vi "ZCAN_FilterClear.vi"(0 "error in (no error)":errorcluster caption="错误输入（无错误）", 2 "can_index_handle":u32, 5 "can_index":u32) -> (14 "error out":errorcluster caption="错误输出", 16 "can_index_handle(out)":u32, 19 "can_index(out)":u32)   [LabVIEW 2020, in "zlgcan.lvlib"]
uses:
  zlgcan.lvlib
  bin/zlgcan_wrap.dll
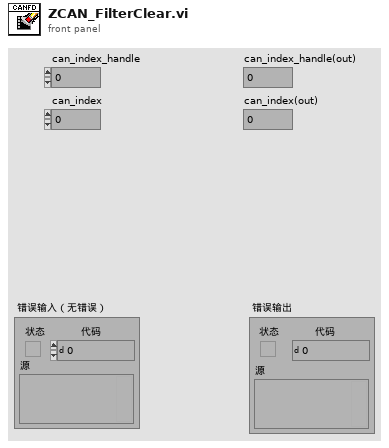
[diagram p1: front panel]
types:
  T1 = cluster{"status":bool, "return":u32, "消息":string}
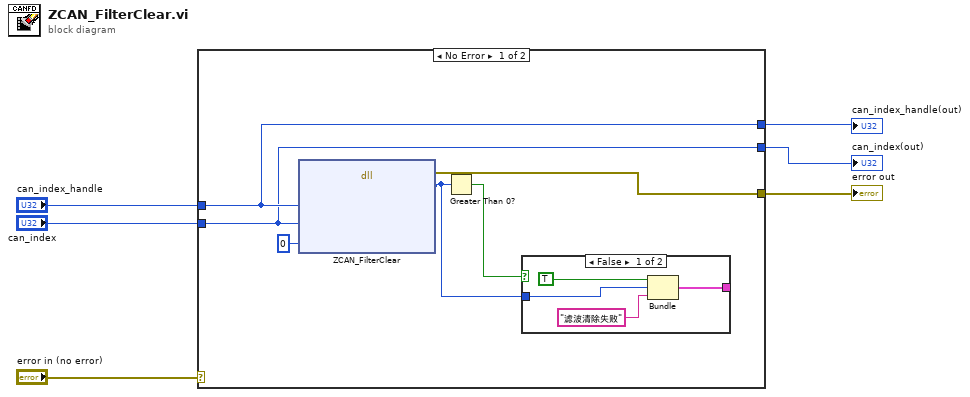
[diagram p0: block diagram]
diagram:
  n1 = case shown="No Error" "error in (no error)" {
    selector: "error in (no error)" -> [_ w17]
    tunnel: [w7 w17] -> w5
    tunnel: "can_index_handle" -> [w10 _]
    tunnel: "can_index" -> [w9 _]
    tunnel: [w10 _] -> w2
    tunnel: [w9 _] -> w1
    frame No Error {
      n2 = dll-call lib="E:/Jabil tools/JabilTestLib/ZLG_CANFD/bin/zlgcan_wrap.dll" fn="ZCAN_FilterClear"("device_handle"=w10, "can_index"=w9, "clear"=0) -> (error out=w7:errorcluster, "return"=w8:u32)  [unwired: 6 in, 1 out]
      n3 = Greater Than 0?(x=w8) -> (x > 0?=w12:bool)
      n4 = case shown="False" w12 {
        tunnel: [w14 _] -> _
        tunnel: w8 -> [w13 _]
        frame False {
          n5 = Bundle("status"=TRUE, "return"=w13, "消息"="滤波清除失败") -> (w14:T1)  [unwired: 1 in]
        }
        frame True {
        }
      }
    }
    frame Error {
    }
  }
  "error out" <- w5
  "can_index_handle(out)" <- w2
  "can_index(out)" <- w1
